vi "test_GetItemInfosFromProjectFile.vi"() -> (3 "Pass?":bool)   [LabVIEW 2019, in "Tests.SolutionBuilder.lvlib"]
uses:
  Tests.SolutionBuilder.lvlib
  SolutionBuilder/SolutionBuilder.lvclass
  SolutionBuilder/ProjectItem/ProjectItem.lvclass
panel:
  out "test results":u32 format="%03b"
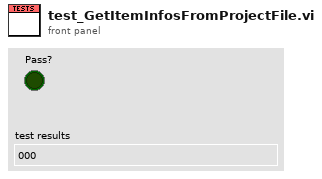
[diagram p1: front panel]
types:
  T1 = typedef "SolutionBuilder.lvlib/SolutionBuilder.lvclass/ProjectItemMap.ctl" = map{path, refnum<class "ProjectItem.lvclass">[]}
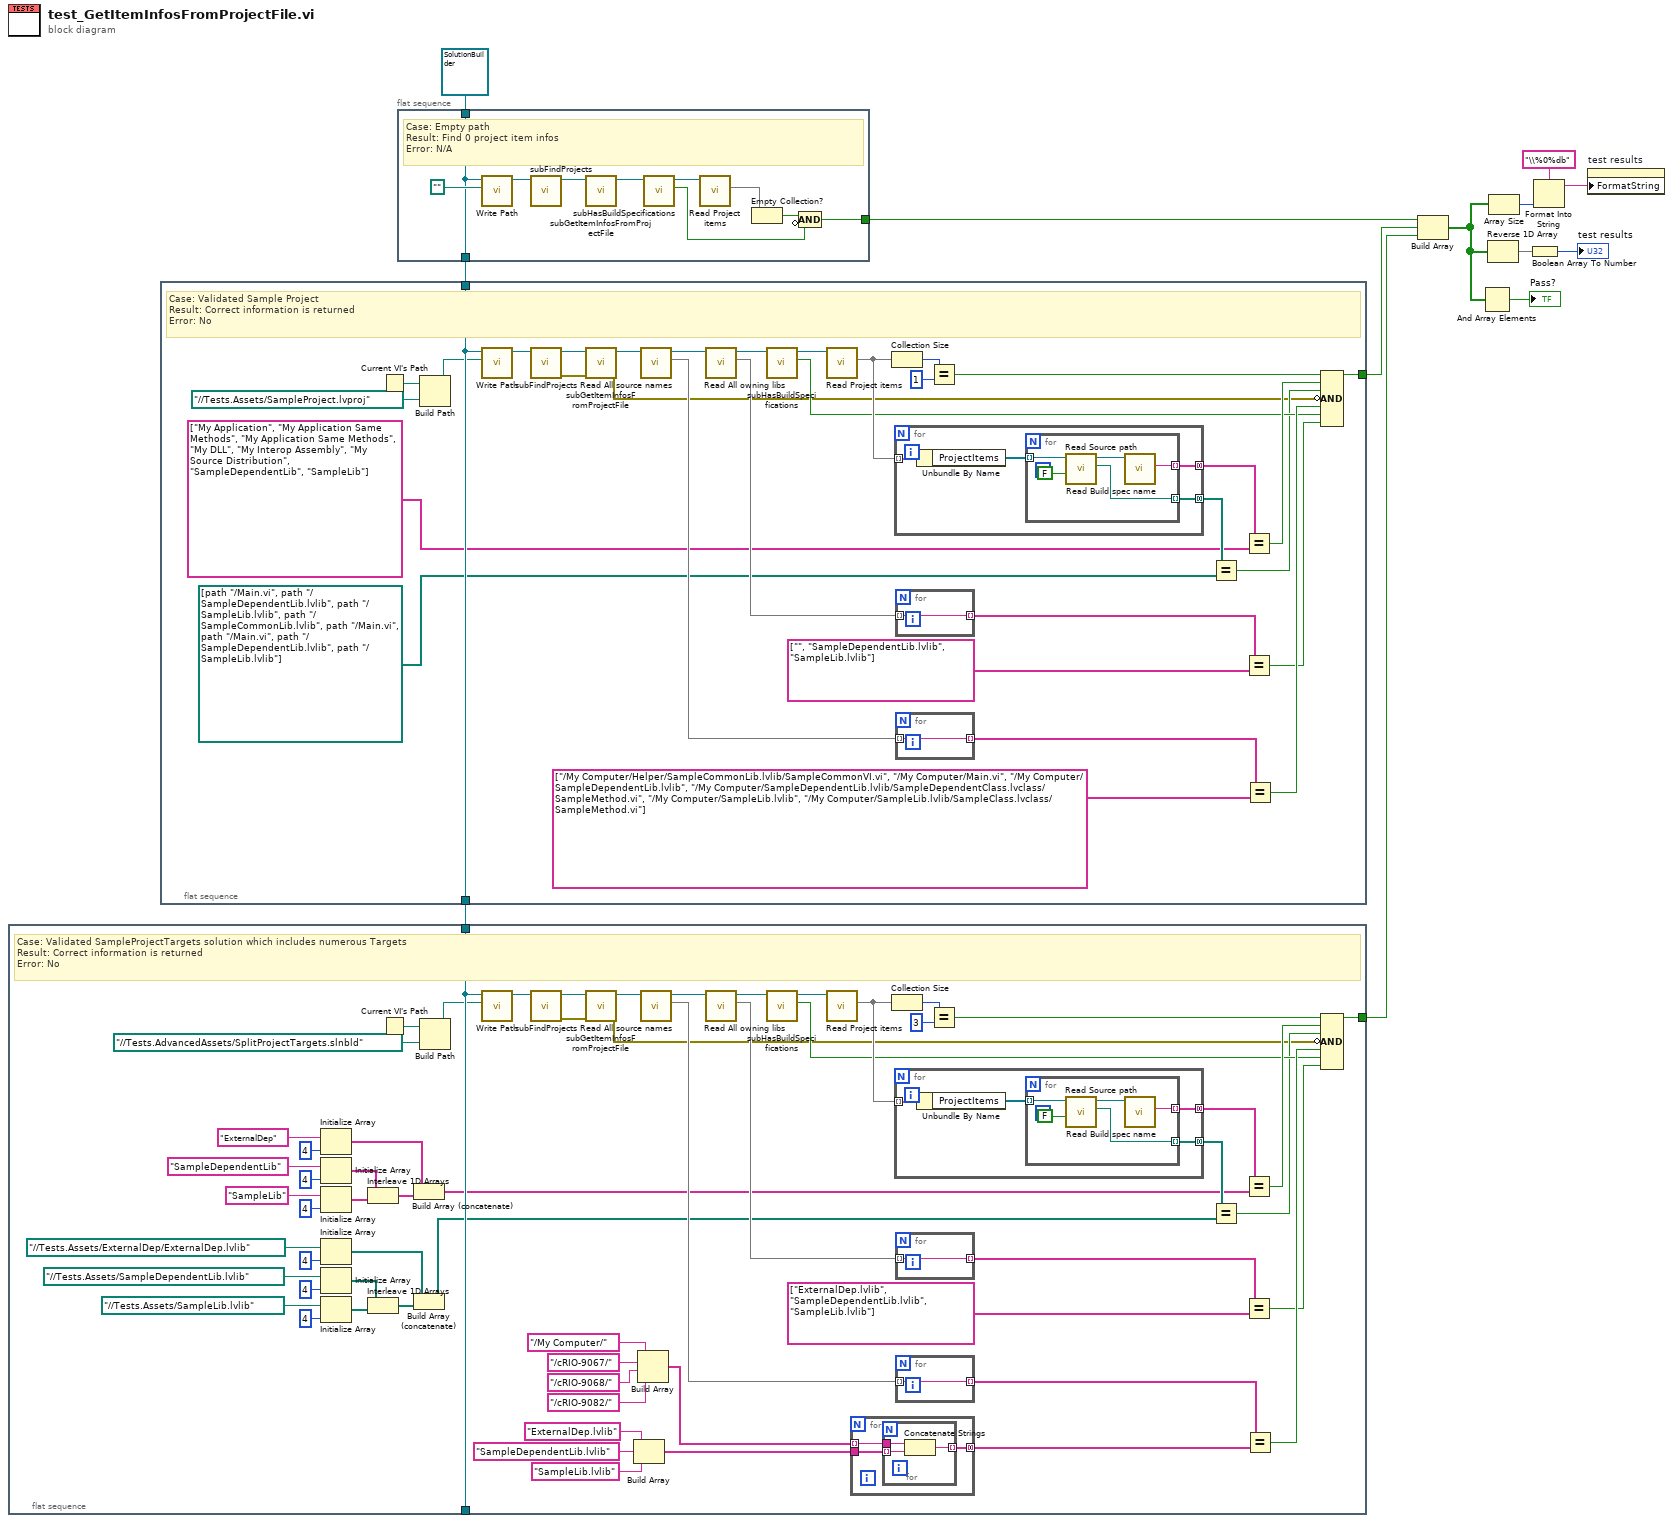
[diagram p0: block diagram]
diagram:
  n1 = flat-sequence {
    tunnel: [w62] -> w1
    tunnel: w2 -> [w73]
    tunnel: [w73] -> _
    frame #0 {
      # "Case: Validated SampleProjectTargets solution which includes numerous Targets\nResult: Correct information is returned\nError: No"
      n2 = Initialize Array("ExternalDep" ("Build spec name"), 4 ("dimension size")) -> (w36:string[])
      n3 = Initialize Array("SampleDependentLib" ("Build spec name"), 4 ("dimension size")) -> (w39:string[])
      n4 = Initialize Array("SampleLib" ("Build spec name"), 4 ("dimension size")) -> (w38:string[])
      n5 = Initialize Array(path "../../Tests.Assets/ExternalDep/ExternalDep.lvlib" ("Source path"), 4 ("dimension size")) -> (w34:path[])
      n6 = Initialize Array(path "../../Tests.Assets/SampleDependentLib.lvlib" ("Source path"), 4 ("dimension size")) -> (w31:path[])
      n7 = Initialize Array(path "../../Tests.Assets/SampleLib.lvlib" ("Source path"), 4 ("dimension size")) -> (w32:path[])
      n8 = Interleave 1D Arrays(w39, w38) -> (w37:string[])
      n9 = Interleave 1D Arrays(w31, w32) -> (w33:path[])
      n10 = Current VI's Path() -> (path=w71:path)
      n11 = Build Array (concatenate)(w36, w37) -> (w35:string[])
      n12 = Build Array (concatenate)(w34, w33) -> (w24:path[])
      n13 = Build Path(base path=w71, name or relative path=path "../../Tests.AdvancedAssets/SplitProjectTargets.slnbld" ("Path")) -> (appended path=w69:path)
      n14 = call-dynamic "Write Path.vi"("Path"=w69, "SolutionBuilder in"=w73) -> ("SolutionBuilder out"=w74:refnum<class "SolutionBuilder.lvclass">)  [unwired: 9 in]
      n15 = call "subFindProjects.vi"("SolutionBuilder in"=w74) -> ("error out"=w47:errorcluster, "SolutionBuilder out"=w72:refnum<class "SolutionBuilder.lvclass">)  [unwired: 9 in]
      n16 = call "subGetItemInfosFromProjectFile.vi"("error in (no error)"=w47, "SolutionBuilder in"=w72) -> ("error out"=w46:errorcluster, "SolutionBuilder out"=w66:refnum<class "SolutionBuilder.lvclass">)  [unwired: 8 in]
      n17 = Build Array("ExternalDep.lvlib" ("Build spec name"), "SampleDependentLib.lvlib" ("Build spec name"), "SampleLib.lvlib" ("Build spec name")) -> (w15:string[])
      n18 = Build Array("/My Computer/" ("Build spec name"), "/cRIO-9067/" ("Build spec name"), "/cRIO-9068/" ("Build spec name"), "/cRIO-9082/" ("Build spec name")) -> (w16:string[])
      n19 = call-dynamic "Read All source names.vi"("SolutionBuilder in"=w66) -> ("All source names"=w61:set{string}, "SolutionBuilder out"=w53:refnum<class "SolutionBuilder.lvclass">)  [unwired: 9 in]
      n20 = call-dynamic "Read All owning libs.vi"("SolutionBuilder in"=w53) -> ("All owning libs"=w51:set{string}, "SolutionBuilder out"=w52:refnum<class "SolutionBuilder.lvclass">)  [unwired: 9 in]
      n21 = call "subHasBuildSpecifications.vi"("SolutionBuilder in"=w52) -> ("Has specs?"=w58:bool, "SolutionBuilder out"=w59:refnum<class "SolutionBuilder.lvclass">)  [unwired: 8 in, 1 out]
      n22 = call-dynamic "Read Project items.vi"("SolutionBuilder in"=w59) -> ("Project items"=w65:T1)  [unwired: 9 in, 1 out]
      n23 = for {
        tunnel: w16 -> [w77] mode=indexing
        tunnel: w15 -> [w76]
        tunnel: [w75] -> w14 mode=concatenating
        n24 = for {
          tunnel: w77 -> [w80]
          tunnel: w76 -> [w79] mode=indexing
          tunnel: [w78] -> w75 mode=indexing
          n25 = Concatenate Strings(w80, w79) -> (w78:string)
        }
      }
      n26 = Collection Size(1:w65) -> (0:w68:i32)
      n27 = for {
        tunnel: w65 -> [w85] mode=indexing
        tunnel: [w84] -> w57 mode=concatenating
        tunnel: [w82] -> w55 mode=concatenating
        n28 = Unbundle By Name(w85) -> ("ProjectItems"=w83:refnum<class "ProjectItem.lvclass">[])
        n29 = for {
          tunnel: w83 -> [w88] mode=indexing
          tunnel: [w90] -> w84 mode=indexing
          tunnel: [w87] -> w82 mode=indexing
          n30 = call-dynamic "Read Source path.vi"("Force abs path? (T)"=FALSE, "ProjectItem in"=w88) -> ("Source path"=w87:path, "ProjectItem out"=w89:refnum<class "ProjectItem.lvclass">)  [unwired: 8 in]
          n31 = call-dynamic "Read Build spec name.vi"("ProjectItem in"=w89) -> ("Build spec name"=w90:string)  [unwired: 9 in, 1 out]
        }
      }
      n32 = for {
        tunnel: w51 -> [w81] mode=indexing
        tunnel: [w81] -> w50 mode=indexing
      }
      n33 = for {
        tunnel: w61 -> [w91] mode=indexing
        tunnel: [w91] -> w56 mode=indexing
      }
      n34 = Equal?(x=w68, y=3) -> (x = y?=w64:bool)
      n35 = Equal?(x=w55, y=w24) -> (x = y?=w54:bool)
      n36 = Equal?(x=w57, y=w35) -> (x = y?=w63:bool)
      n37 = Equal?(x=w50, y=string[] ["ExternalDep.lvlib", "SampleDependentLib.lvlib", "SampleLib.lvlib"] ("Array")) -> (x = y?=w48:bool)
      n38 = Equal?(x=w56, y=w14) -> (x = y?=w60:bool)
      n39 = Compound Arithmetic op=AND(w64, w63, w54, invert w46, w60, w58, w48) -> (w62:bool)
    }
  }
  n40 = flat-sequence {
    tunnel: [w111] -> w4
    tunnel: w5 -> [w122]
    tunnel: [w122] -> w2
    frame #0 {
      # "Case: Validated Sample Project\nResult: Correct information is returned\nError: No"
      n41 = Current VI's Path() -> (path=w120:path)
      n42 = Build Path(base path=w120, name or relative path=path "../../Tests.Assets/SampleProject.lvproj" ("Path")) -> (appended path=w118:path)
      n43 = call-dynamic "Write Path.vi"("Path"=w118, "SolutionBuilder in"=w122) -> ("SolutionBuilder out"=w123:refnum<class "SolutionBuilder.lvclass">)  [unwired: 9 in]
      n44 = call "subFindProjects.vi"("SolutionBuilder in"=w123) -> ("error out"=w93:errorcluster, "SolutionBuilder out"=w121:refnum<class "SolutionBuilder.lvclass">)  [unwired: 9 in]
      n45 = call "subGetItemInfosFromProjectFile.vi"("error in (no error)"=w93, "SolutionBuilder in"=w121) -> ("error out"=w92:errorcluster, "SolutionBuilder out"=w115:refnum<class "SolutionBuilder.lvclass">)  [unwired: 8 in]
      n46 = call-dynamic "Read All source names.vi"("SolutionBuilder in"=w115) -> ("All source names"=w110:set{string}, "SolutionBuilder out"=w101:refnum<class "SolutionBuilder.lvclass">)  [unwired: 9 in]
      n47 = call-dynamic "Read All owning libs.vi"("SolutionBuilder in"=w101) -> ("All owning libs"=w99:set{string}, "SolutionBuilder out"=w100:refnum<class "SolutionBuilder.lvclass">)  [unwired: 9 in]
      n48 = call "subHasBuildSpecifications.vi"("SolutionBuilder in"=w100) -> ("Has specs?"=w107:bool, "SolutionBuilder out"=w108:refnum<class "SolutionBuilder.lvclass">)  [unwired: 8 in, 1 out]
      n49 = call-dynamic "Read Project items.vi"("SolutionBuilder in"=w108) -> ("Project items"=w114:T1)  [unwired: 9 in, 1 out]
      n50 = Collection Size(1:w114) -> (0:w117:i32)
      n51 = for {
        tunnel: w114 -> [w128] mode=indexing
        tunnel: [w127] -> w106 mode=concatenating
        tunnel: [w125] -> w103 mode=concatenating
        n52 = Unbundle By Name(w128) -> ("ProjectItems"=w126:refnum<class "ProjectItem.lvclass">[])
        n53 = for {
          tunnel: w126 -> [w131] mode=indexing
          tunnel: [w133] -> w127 mode=indexing
          tunnel: [w130] -> w125 mode=indexing
          n54 = call-dynamic "Read Source path.vi"("Force abs path? (T)"=FALSE, "ProjectItem in"=w131) -> ("Source path"=w130:path, "ProjectItem out"=w132:refnum<class "ProjectItem.lvclass">)  [unwired: 8 in]
          n55 = call-dynamic "Read Build spec name.vi"("ProjectItem in"=w132) -> ("Build spec name"=w133:string)  [unwired: 9 in, 1 out]
        }
      }
      n56 = for {
        tunnel: w99 -> [w124] mode=indexing
        tunnel: [w124] -> w98 mode=indexing
      }
      n57 = for {
        tunnel: w110 -> [w134] mode=indexing
        tunnel: [w134] -> w105 mode=indexing
      }
      n58 = Equal?(x=w117, y=1) -> (x = y?=w113:bool)
      n59 = Equal?(x=w103, y=path[] [path "../Main.vi", path "../SampleDependentLib.lvlib", path "../SampleLib.lvlib", path "../SampleCommonLib.lvlib", path "../Main.vi", path "../Main.vi", path "../SampleDependentLib.lvlib", path "../SampleLib.lvlib"] ("Array 2")) -> (x = y?=w102:bool)
      n60 = Equal?(x=w106, y=string[] ["My Application", "My Application Same Methods", "My Application Same Methods", "My DLL", "My Interop Assembly", "My Source Distribution", "SampleDependentLib", "SampleLib"] ("Array")) -> (x = y?=w112:bool)
      n61 = Equal?(x=w98, y=string[] ["", "SampleDependentLib.lvlib", "SampleLib.lvlib"] ("Array")) -> (x = y?=w96:bool)
      n62 = Equal?(x=w105, y=string[] ["/My Computer/Helper/SampleCommonLib.lvlib/SampleCommonVI.vi", "/My Computer/Main.vi", "/My Computer/SampleDependentLib.lvlib", "/My Computer/SampleDependentLib.lvlib/SampleDependentClass.lvclass/SampleMethod.vi", "/My Computer/SampleLib.lvlib", "/My Computer/SampleLib.lvlib/SampleClass.lvclass/SampleMethod.vi"] ("Array 2")) -> (x = y?=w109:bool)
      n63 = Compound Arithmetic op=AND(w113, w112, w102, invert w92, w109, w107, w96) -> (w111:bool)
    }
  }
  n64 = flat-sequence {
    tunnel: [w135] -> w7
    tunnel: refnum<class "SolutionBuilder.lvclass"> refnum ("SolutionBuilder in") -> [w142]
    tunnel: [w142] -> w5
    frame #0 {
      # "Case: Empty path\nResult: Find 0 project item infos\nError: N/A"
      n65 = call-dynamic "Write Path.vi"("Path"=path "", "SolutionBuilder in"=w142) -> ("SolutionBuilder out"=w144:refnum<class "SolutionBuilder.lvclass">)  [unwired: 9 in]
      n66 = call "subFindProjects.vi"("SolutionBuilder in"=w144) -> ("SolutionBuilder out"=w141:refnum<class "SolutionBuilder.lvclass">)  [unwired: 9 in, 1 out]
      n67 = call "subGetItemInfosFromProjectFile.vi"("SolutionBuilder in"=w141) -> ("SolutionBuilder out"=w138:refnum<class "SolutionBuilder.lvclass">)  [unwired: 9 in, 1 out]
      n68 = call "subHasBuildSpecifications.vi"("SolutionBuilder in"=w138) -> ("Has specs?"=w136:bool, "SolutionBuilder out"=w137:refnum<class "SolutionBuilder.lvclass">)  [unwired: 8 in, 1 out]
      n69 = call-dynamic "Read Project items.vi"("SolutionBuilder in"=w137) -> ("Project items"=w140:T1)  [unwired: 9 in, 1 out]
      n70 = Empty Collection?(1:w140) -> (0:w139:bool)
      n71 = Compound Arithmetic op=AND(w139, invert w136) -> (w135:bool)
    }
  }
  n72 = Build Array(w7, w4, w1) -> (w11:bool[])
  n73 = And Array Elements(Boolean array=w11) -> (logical AND=→"Pass?":bool)
  n74 = Reverse 1D Array(array=w11) -> (reversed array=w3:bool[])
  n75 = Array Size(array=w11) -> (size(s)=w9:i32)
  n76 = Boolean Array To Number(Boolean array=w3) -> (number=→"test results":u32)
  n77 = Format Into String(format string="\\%0%db", w9) -> (resulting string=w8:string)  [unwired: 2 in, 1 out]
  n78 = property on="test results" class="DigNum (strict)"("FormatString"=w8) -> ()  [unwired: 2 in, 2 out]
